vi "Get TaskRef from TaskID.vi"(8 "error in (no error)":errorcluster, 10 "TaskID":string) -> (0 "error out":errorcluster, 2 "IO Task.Task Ref":refnum<k21>)   [LabVIEW 2020, in "DAQDict.lvlib"]
uses:
  DAQDict.lvlib
  support/IO Task--cluster.ctl
  support/IO Task Dict Node--cluster.ctl
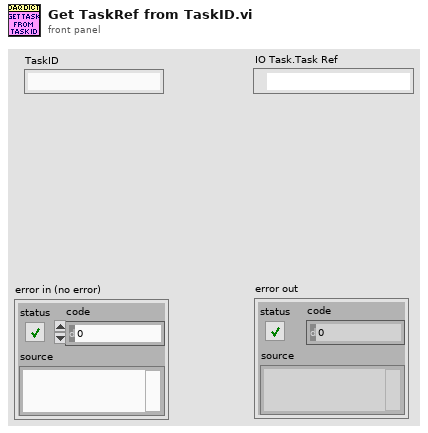
[diagram p1: front panel]
types:
  T1 = typedef "IO Task Dict Node--cluster.ctl" = cluster{"IO Type":enum16{"N/A", "DI", "DO"}, "IONames":string[], "values":bool[], "IO Task":T2}
  T2 = typedef "IO Task--cluster.ctl" = cluster{"IO Type":enum16{"N/A", "DI", "DO"}, "TaskID":string, "IONames":string[], "ChPath":string[], "Task Ref":refnum<k21>}
  T3 = typedef "TD Dynamic CVT DVR--ref.ctl" = refnum<data-value>
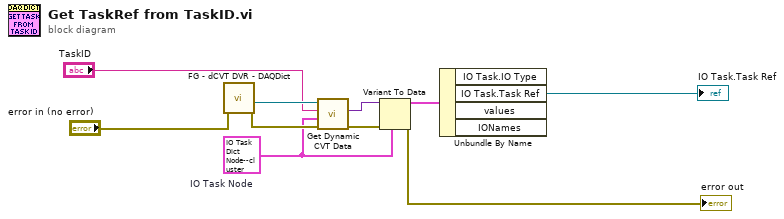
[diagram p0: block diagram]
diagram:
  w4 = T1 {"IO Type"=enum."N/A", "IONames"=[], "values"=[], "IO Task"={"IO Type"=enum."N/A", "TaskID"="", "IONames"=[], "ChPath"=[], "Task Ref"=""}}  # IO Task Node
  n1 = call "FG - dCVT DVR - DAQDict.vi"("error in (no error)"="error in (no error)") -> ("dCVT DAQDict out"=w8:T3, "error out"=w10:errorcluster)  [unwired: 8 in]
  n2 = call <vilib>:"Get Dynamic CVT Data.vi"("error in (no error)"=w10, "default value (empty variant)"=w4, "DataName"="TaskID", "dCVT DVR"=w8) -> ("error out"=w9:errorcluster, "value"=w5:variant)  [unwired: 4 in, 2 out]
  n3 = Variant To Data(error in=w9, type=w4, Variant=w5) -> (data=w3:T1, error out=→"error out":errorcluster)
  n4 = Unbundle By Name(w3) -> ("IO Task.Task Ref"=→"IO Task.Task Ref":refnum<k21>)  [unwired: 3 out]
